vi "GetExtensionInfo.vi"(8 "error in (no error)":errorcluster, 11 "Zero Offset and Degree Transitions in":refnum<class "Zero Offset and Degree Transitions.lvclass">) -> (0 "error out":errorcluster, 2 "Extension Info":T1, 3 "Zero Offset and Degree Transitions out":refnum<class "Zero Offset and Degree Transitions.lvclass">)   [LabVIEW 2013, in "File Formats.lvlib" / "Zero Offset and Degree Transitions.lvclass"]
uses:
  Zero Offset and Degree Transitions.lvclass
  Parent/Extension Info.ctl
  Parent/FileFormat.lvclass
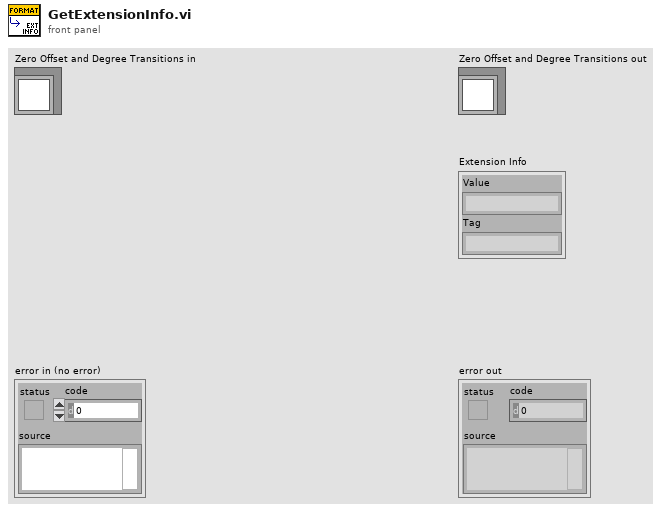
[diagram p1: front panel]
types:
  T1 = typedef "File Formats.lvlib/FileFormat.lvclass/Extension Info.ctl" = cluster{"Value":string, "Tag":string}
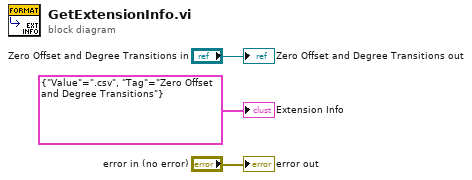
[diagram p0: block diagram]
diagram:
  "error out" <- "error in (no error)"
  "Zero Offset and Degree Transitions out" <- "Zero Offset and Degree Transitions in"
  "Extension Info" <- T1 {"Value"=".csv", "Tag"="Zero Offset and Degree Transitions"} ("Extension Info")
